vi "get_value_type.vi"(8 "error in (no error)":errorcluster, 11 "Value in":refnum<class "Value.lvclass">) -> (0 "error out":errorcluster, 2 "value_type":T1, 3 "Value out":refnum<class "Value.lvclass">)   [LabVIEW 2020, in "toml_edit.lvlib" / "Value.lvclass"]
uses:
  Value.lvclass
  value_type--enum.ctl
  Value.lvclass/Value.ctl
  toml_edit.lvlib
  dragon_toml_64.dll
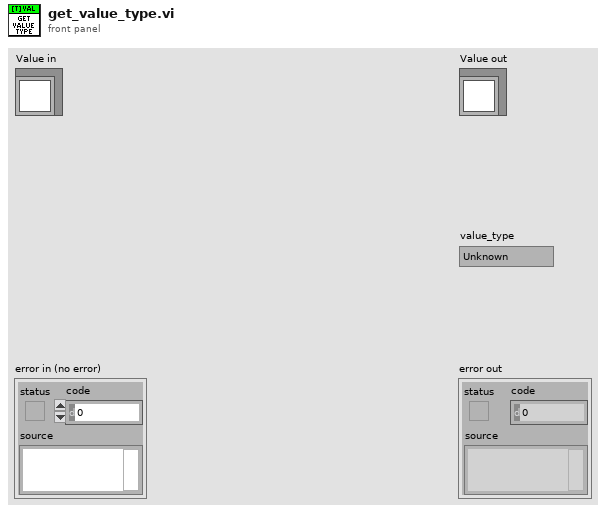
[diagram p1: front panel]
types:
  T1 = typedef "toml_edit.lvlib/Value.lvclass/value_type--enum.ctl" = enum16{"Unknown", "String", "Integer", "Float", "Boolean", "Datetime", "Array", "InlineTable"}
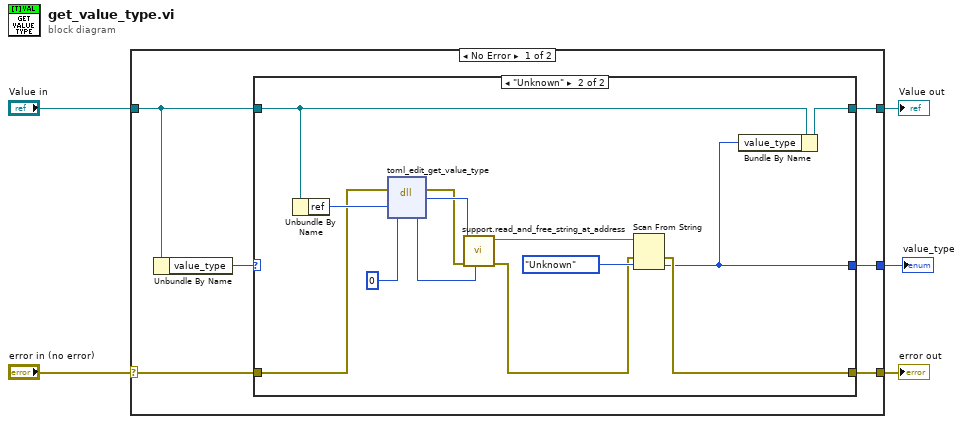
[diagram p0: block diagram]
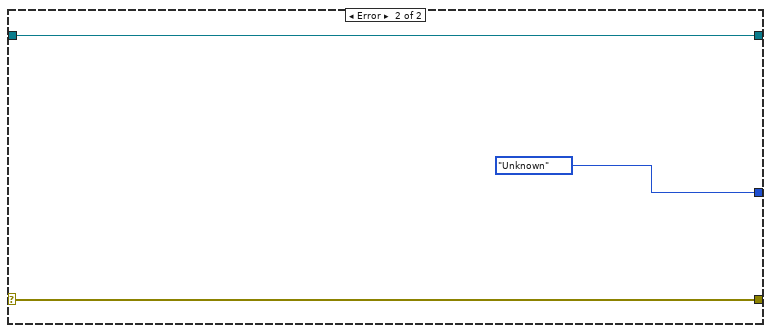
[diagram p3: hidden frame]
diagram:
  n1 = case shown="No Error" "error in (no error)" {
    selector: "error in (no error)" -> [w11 w30]
    tunnel: [w10 w30] -> w4
    tunnel: [w9 w29] -> w2
    tunnel: "Value in" -> [w7 w29]
    tunnel: [w8 value_type--enum."Unknown" ("type")] -> w1
    frame No Error {
      n2 = Unbundle By Name(w7) -> ("value_type"=w6:T1)
      n3 = case shown="\"Unknown\"" w6 {
        selector: w6 -> [w14 _]
        tunnel: w7 -> [w12 w23]
        tunnel: w11 -> [w13 w22]
        tunnel: [w13 w20] -> w10
        tunnel: [w12 w18] -> w9
        tunnel: [w14 w17] -> w8
        frame Default {
        }
        frame "Unknown" {
          n4 = Unbundle By Name(w23) -> ("ref"=w25:u64)
          n5 = dll-call lib="C:/projects/dragon-desktop/source/submodules/toml-edit-labview/lv_src/dragon_toml_*.*" fn="toml_edit_get_value_type"(error in=w22, "item_ref"=w25, "string_length"=u32 0) -> (error out=w26:errorcluster, "string_ptr"=w27:u64, "string_length"=w16:u32)  [unwired: 3 in, 1 out]
          n6 = call "support.read_and_free_string_at_address.vi"("string_length"=w16, "error in (no error)"=w26, "string_ptr"=w27) -> ("error out"=w21:errorcluster, "string"=w19:string)  [unwired: 7 in]
          n7 = Scan From String(input string=w19, error in=w21, default 1=value_type--enum."Unknown" ("type")) -> (error out=w20:errorcluster, output 1=w17:T1)  [unwired: 2 in, 2 out]
          n8 = Bundle By Name(cluster=w23, "value_type"=w17) -> (w18:refnum<class "Value.lvclass">)
        }
      }
    }
    frame Error {
    }
  }
  "error out" <- w4
  "Value out" <- w2
  "value_type" <- w1
